vi "Untitled 2.vi"   [LabVIEW 2020]
uses:
  <vilib>/Instr/_visa.llb/VISA Flush IO Buffer Mask.ctl
  <vilib>/Instr/_visa.llb/VISA Configure Serial Port (Instr).vi
types:
  T1 = typedef "VISA Flush IO Buffer Mask.ctl" = u16
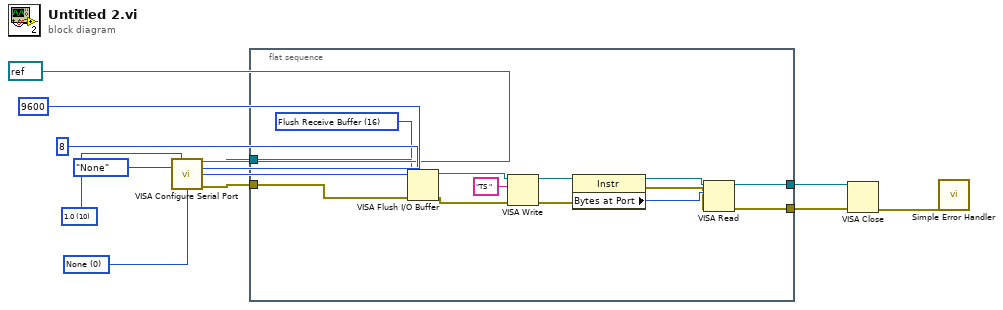
[diagram p0: block diagram]
diagram:
  w6 = u16 0 items=["None", "XON/XOFF", "RTS/CTS", "XON/XOFF & RTS/CTS", "DTR/DSR", "XON/XOFF & DTR/DSR"] ("flow control (0:none)")
  w7 = u16 10 items=["1.0"=10, "1.5"=15, "2.0"=20] ("stop bits (10: 1 bit)")
  n1 = call-poly "VISA Configure Serial Port"("VISA resource name"=refnum<visa-resource-name> refnum, "baud rate (9600)"=u32 9600, "data bits (8)"=u16 8, "parity (0:none)"=enum16{"None", "Odd", "Even", "Mark", "Space"}."None", "stop bits (10: 1 bit)"=w7, "flow control (0:none)"=w6) -> ("VISA resource name out"=w5:refnum<visa-resource-name>, "error out"=w4:errorcluster)  [unwired: 8 in]
  n2 = flat-sequence {
    tunnel: w5 -> [w24]
    tunnel: w4 -> [w23]
    tunnel: [w13] -> w3
    tunnel: [w12] -> w2
    frame #0 {
      w22 = T1 16 items=["Flush Receive Buffer"=16, "Write Transmit Buffer to Device"=32, "Flush Receive Buffer (No I/O)"=64, "Flush Transmit Buffer"=128] ("Mask")
      n3 = VISA Flush I/O Buffer(VISA resource name=w24, mask (16)=w22, error in (no error)=w23) -> (VISA resource name out=w20:refnum<visa-resource-name>, error out=w19:errorcluster)
      n4 = VISA Write(VISA resource name=w20, write buffer="TS ", error in (no error)=w19) -> (VISA resource name out=w18:refnum<visa-resource-name>, error out=w17:errorcluster)  [unwired: 1 out]
      n5 = property class="Instr"(reference=w18, error in=w17) -> (reference out=w16:refnum<visa-resource-name>, error out=w14:errorcluster, "Bytes at Port"=w15:u32)
      n6 = VISA Read(VISA resource name=w16, byte count=w15, error in (no error)=w14) -> (VISA resource name out=w12:refnum<visa-resource-name>, error out=w13:errorcluster)  [unwired: 2 out]
    }
  }
  n7 = VISA Close(VISA resource name=w2, error in (no error)=w3) -> (error out=w1:errorcluster)
  n8 = call <vilib>:"Simple Error Handler.vi"("error in (no error)"=w1) -> ()  [unwired: 4 in, 5 out]
